vi "Init Telemetry.vi"(8 "error in (no error)":errorcluster, 11 "Application in":refnum<class "Application.lvclass">) -> (0 "error out":errorcluster, 3 "Application out":refnum<class "Application.lvclass">)   [LabVIEW 2023, in "Application.lvlib" / "Application.lvclass"]
uses:
  Application.lvclass
  <vilib>/Utility/error.llb/Trim Whitespace One-Sided.vi
  Application.lvclass/Application.ctl
  <vilib>/Utility/config.llb/Read Key (Boolean).vi
  <vilib>/httpClient/POSTBuffer.vi
  <vilib>/Utility/config.llb/Write Key (String).vi
  <vilib>/Utility/config.llb/Read Key (String).vi
  <vilib>/httpClient/LabVIEWHTTPClient.lvlib
  <vilib>/Utility/config.llb/NI_LVConfig.lvlib
  Application.lvlib
panel:
  out "reply body":string
  out "reply headers":string
  out "JSON to server":string
  out "HTTP error":errorcluster
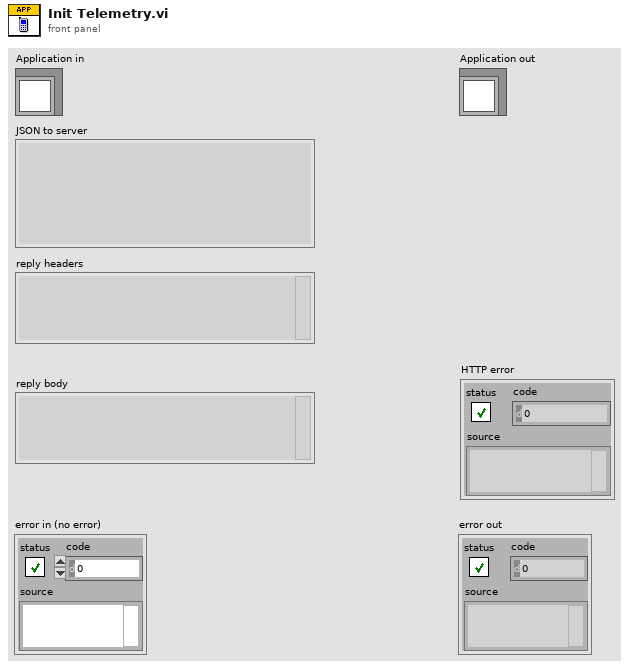
[diagram p1: front panel]
types:
  T1 = cluster{"api_key":string, "event":string, "distinct_id":string, "properties":cluster{"app_version":string, "OS":string}}
  T2 = typedef "NI_LVConfig.lvlib/Config Data RefNum.ctl" = refnum<k1>
  T3 = typedef "LabVIEWHTTPClient.lvlib/ClientHandle.ctl" = refnum<k1>
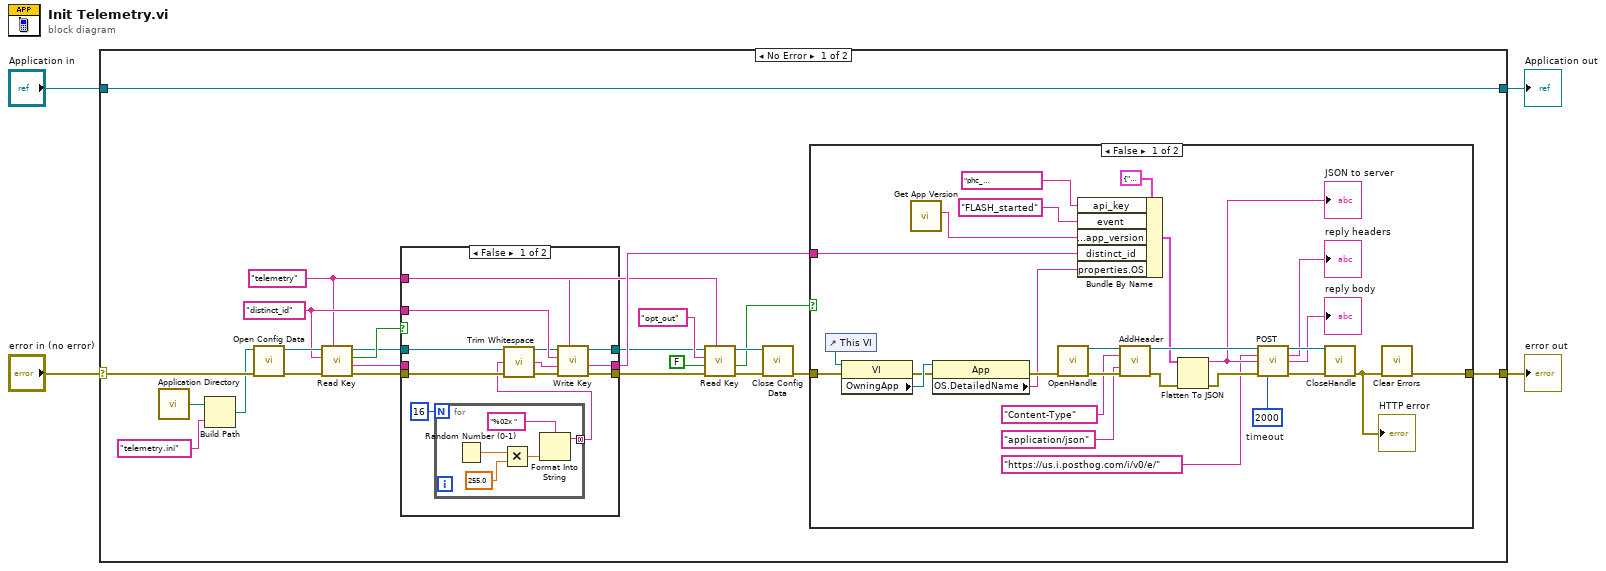
[diagram p0: block diagram]
diagram:
  n1 = case shown="No Error" "error in (no error)" {
    selector: "error in (no error)" -> [w26 w75]
    tunnel: [w27 w75] -> w3
    tunnel: [w5 w74] -> w1
    tunnel: "Application in" -> [w5 w74]
    frame No Error {
      w8 = "telemetry" ("key")
      w17 = "distinct_id" ("key")
      n2 = call <vilib>:"Application Directory.vi"() -> ("Application Directory"=w16:path)
      n3 = Build Path(base path=w16, name or relative path="telemetry.ini" ("key")) -> (appended path=w14:path)
      n4 = call <vilib>:"Open Config Data.vi"("error in (no error)"=w26, "configuration file path"=w14) -> ("error out"=w25:errorcluster, "refnum"=w24:T2)  [unwired: 7 in, 1 out]
      n5 = call-poly <vilib>:"Read Key.vi"("section"=w8, "error in (no error)"=w25, "key"=w17, "refnum"=w24) -> ("error out"=w21:errorcluster, "value"=w19:string, "found?"=w22:bool, "refnum out"=w20:T2)  [unwired: 4 in]
      n6 = case shown="False" w22 {
        tunnel: w21 -> [w36 w44]
        tunnel: [w35 w44] -> w6
        tunnel: w20 -> [w33 w43]
        tunnel: [w32 w43] -> w7
        tunnel: w19 -> [_ w42]
        tunnel: [w30 w42] -> w18
        tunnel: w17 -> [w34 _]
        tunnel: w8 -> [w28 _]
        frame False {
          n7 = for {
            N: 16 -> [_]
            tunnel: [w38] -> w29 mode=concatenating
            n8 = Random Number (0-1)() -> (number: 0 to 1=w41:dbl)
            n9 = Multiply(x=w41, y=255.0) -> (x*y=w39:dbl)
            n10 = Format Into String(format string="%02x ", w39) -> (resulting string=w38:string)  [unwired: 2 in, 1 out]
          }
          n11 = call <vilib>:"Trim Whitespace.vi"("string"=w29) -> ("trimmed string"=w30:string)  [unwired: 1 in]
          n12 = call-poly <vilib>:"Write Key.vi"("section"=w28, "error in (no error)"=w36, "value"=w30, "key"=w34, "refnum"=w33) -> ("error out"=w35:errorcluster, "refnum out"=w32:T2)  [unwired: 4 in, 1 out]
        }
        frame True {
          # "Use existing ID"
        }
      }
      n13 = call-poly <vilib>:"Read Key.vi"("section"=w8, "error in (no error)"=w6, "default value"=FALSE, "key"="opt_out", "refnum"=w7) -> ("error out"=w12:errorcluster, "value"=w10:bool, "refnum out"=w13:T2)  [unwired: 3 in, 1 out]
      n14 = call <vilib>:"Close Config Data.vi"("error in (no error)"=w12, "refnum"=w13) -> ("error out"=w23:errorcluster)  [unwired: 8 in, 1 out]
      n15 = case shown="False" w10 {
        tunnel: [w70 w73] -> w27
        tunnel: w23 -> [w52 w73]
        tunnel: w18 -> [w51 _]
        frame False {
          w63 = 2000  # timeout
          n16 = control-ref of="This VI"() -> (w56:refnum<vi>)
          n17 = property class="VI"(reference=w56, error in=w52) -> (error out=w54:errorcluster, "OwningApp"=w55:refnum<vi>)  [unwired: 1 out]
          n18 = call "Get App Version.vi"() -> ("String"=w45:string)  [unwired: 10 in, 1 out]
          n19 = property class="App"(reference=w55, error in=w54) -> (error out=w53:errorcluster, "OS.DetailedName"=w46:string)  [unwired: 1 out]
          n20 = call <vilib>:"OpenHandle.vi"("error in (no error)"=w53) -> ("client handle out"=w67:T3, "error out"=w68:errorcluster)  [unwired: 13 in]
          n21 = Bundle By Name(cluster=T1 {"api_key"="", "event"="", "distinct_id"="", "properties"={"app_version"="", "OS"=""}} ("posthog_POST"), "api_key"="phc_cpOjVvNuHOKGji8EFCs9hGCKToPLYCe960qFAamlI20", "event"="FLASH_started", "properties.app_version"=w45, "distinct_id"=w51, "properties.OS"=w46) -> (w58:T1)
          n22 = call <vilib>:"AddHeader.vi"("client handle"=w67, "header"="Content-Type", "value"="application/json", "error in (no error)"=w68) -> ("client handle out"=w66:T3, "error out"=w62:errorcluster)  [unwired: 10 in]
          n23 = Flatten To JSON(anything=w58, error in (no error)=w62) -> (JSON string=w60:string, 11:w61:errorcluster)  [unwired: 1 in]
          "JSON to server" <- w60
          n24 = call-poly <vilib>:"POST.vi"("client handle"=w66, "url"="https://us.i.posthog.com/i/v0/e/", "buffer"=w60, "error in (no error)"=w61, "timeout (10000)"=w63) -> ("client handle out"=w69:T3, "headers"=→"reply headers":string, "body"=→"reply body":string, "error out"=w72:errorcluster)  [unwired: 7 in]
          n25 = call <vilib>:"CloseHandle.vi"("client handle"=w69, "error in (no error)"=w72) -> ("error out"=w71:errorcluster)  [unwired: 13 in]
          "HTTP error" <- w71
          n26 = call <vilib>:"Clear Errors.vi"("error in (no error)"=w71) -> ("error out"=w70:errorcluster)  [unwired: 5 in, 1 out]
        }
        frame True {
          # "out out of all telemetry"
        }
      }
    }
    frame Error {
    }
  }
  "error out" <- w3
  "Application out" <- w1
